vi "Send to Server.vi"() -> ()   [LabVIEW 2016]
uses:
  AE Data.ctl
  Array AE Data.ctl
  <vilib>/httpClient/POSTBuffer.vi
  <vilib>/Utility/error.llb/Error Cluster From Error Code.vi
  <vilib>/ErrorRing/Error Ring.xnode
  <vilib>/httpClient/LabVIEWHTTPClient.lvlib
panel:
  out "error out 2":errorcluster
  in  "Tab Control":enum32{"Update My Details", "Debug"}(tab)
  in  "STOP":bool
  in  "Update":bool
  in  "AE":T1
  out "error out":errorcluster
  out "Array of AEs":T2=[{"Name"="Peng", "Go?"=TRUE, "Which batch?"=enum."Anything"}, {"Name"="Xue Sheng", "Go?"=TRUE, "Which batch?"=enum."Anything"}, {"Name"="Denny", "Go?"=TRUE, "Which batch?"=enum."Anything"}, {"Name"="Wilbur", "Go?"=TRUE, "Which batch?"=enum."Anything"}, {"Name"="Hafiz", "Go?"=TRUE, "Which batch?"=enum."Anything"}, {"Name"="James", "Go?"=TRUE, "Which batch?"=enum."Anything"}, {"Name"="Sharath", "Go?"=TRUE, "Which batch?"=enum."Anything"}, {"Name"="Habib", "Go?"=TRUE, "Which batch?"=enum."Anything"}, {"Name"="Stephen", "Go?"=TRUE, "Which batch?"=enum."Anything"}]
  in  "Get List":bool
  in  "url":string="http://10.155.16.37:8002/AELunch/Send"
  out "body":string
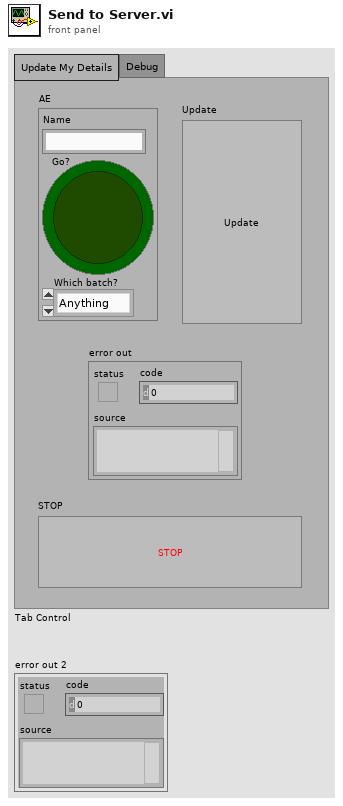
[diagram p1: front panel]
types:
  T1 = typedef "AE Data.ctl" = cluster{"Name":string, "Go?":bool, "Which batch?":enum16{"Anything", "First", "Second"}}
  T2 = typedef "Array AE Data.ctl" = T1[]
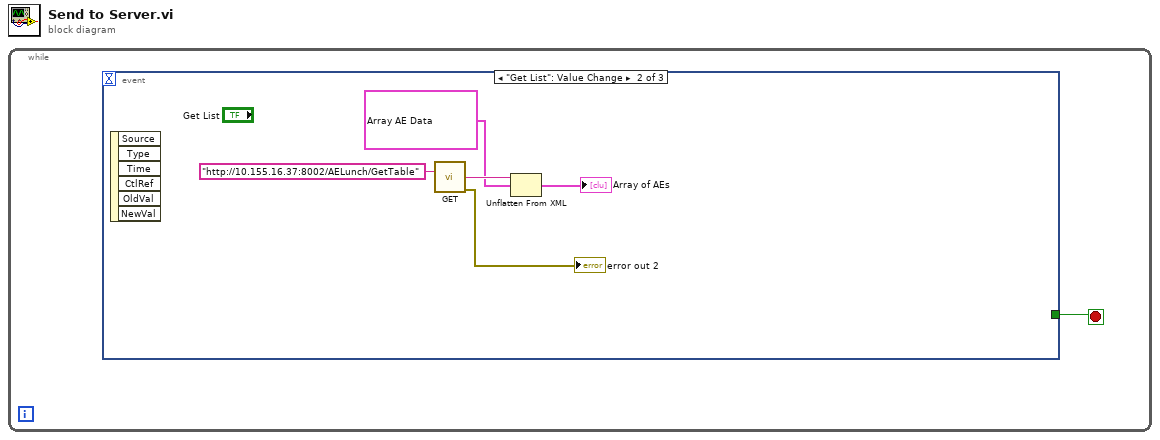
[diagram p0: block diagram]
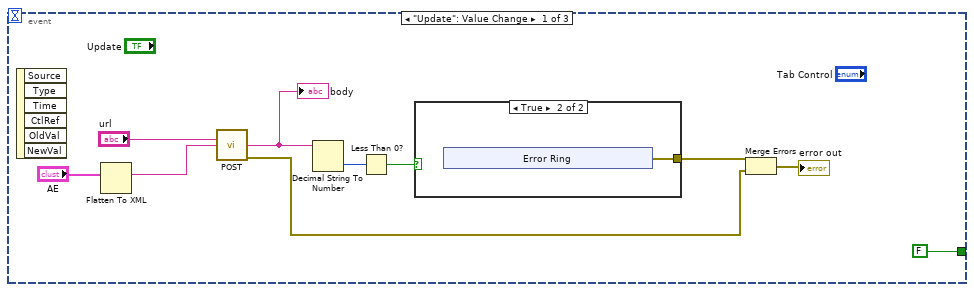
[diagram p2: hidden frame]
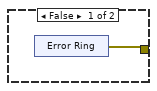
[diagram p3: hidden frame]
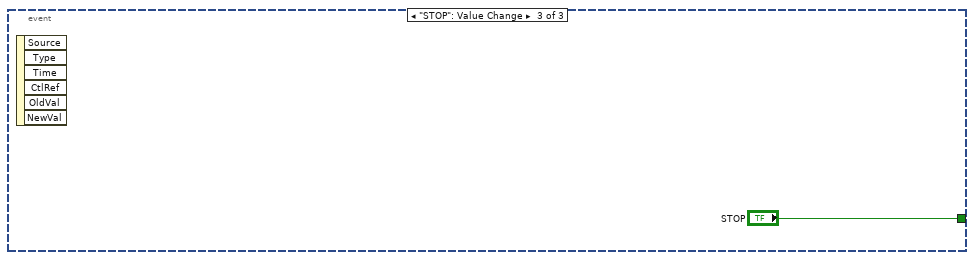
[diagram p4: hidden frame]
diagram:
  n1 = while {
    stop <- w1 stop-if-true
    n2 = event shown="[1] \"Get List\": Value Change" {
      selector: _ -> [_ _ _]
      dyn-events: _ -> [_ _ _]
      timeout: _ -> [_ _ _]
      tunnel: [FALSE _ "STOP"] -> w1
      event "Update": Value Change {
        n3 = event-data() -> ()  [unwired: 1 in, 6 out]
        n4 = Flatten To XML(anything="AE") -> (xml string=w9:string)
        n5 = call-poly <vilib>:"POST.vi"("url"="url", "buffer"=w9) -> ("body"=w8:string, "error out"=w4:errorcluster)  [unwired: 10 in, 2 out]
        "body" <- w8
        n6 = Decimal String To Number(string=w8) -> (number=w7:i32)  [unwired: 2 in, 1 out]
        n7 = Less Than 0?(x=w7) -> (x < 0?=w6:bool)
        n8 = case shown="True" w6 {
          tunnel: [w12 w14] -> w5
          frame False {
            n9 = xnode "Error Ring"() -> ("error out"=w12:errorcluster)
          }
          frame True {
            n10 = xnode "Error Ring"() -> ("error out"=w14:errorcluster)
          }
        }
        n11 = Merge Errors(w5, w4) -> (→"error out":errorcluster)
      }
      event "Get List": Value Change {
        n12 = event-data() -> ()  [unwired: 1 in, 6 out]
        n13 = call <vilib>:"GET.vi"("url"="http://10.155.16.37:8002/AELunch/GetTable") -> ("body"=w23:string, "error out"=→"error out 2":errorcluster)  [unwired: 11 in, 2 out]
        n14 = Unflatten From XML(xml string=w23, type=T2 [{"Name"="Peng", "Go?"=TRUE, "Which batch?"=enum."Anything"}, {"Name"="Xue Sheng", "Go?"=TRUE, "Which batch?"=enum."Anything"}, {"Name"="Denny", "Go?"=TRUE, "Which batch?"=enum."Anything"}, {"Name"="Wilbur", "Go?"=TRUE, "Which batch?"=enum."Anything"}, {"Name"="Hafiz", "Go?"=TRUE, "Which batch?"=enum."Anything"}, {"Name"="James", "Go?"=TRUE, "Which batch?"=enum."Anything"}, {"Name"="Sharath", "Go?"=TRUE, "Which batch?"=enum."Anything"}, {"Name"="Habib", "Go?"=TRUE, "Which batch?"=enum."Anything"}, {"Name"="Stephen", "Go?"=TRUE, "Which batch?"=enum."Anything"}] ("Array of AEs 2")) -> (value=→"Array of AEs":T2)  [unwired: 1 in, 1 out]
      }
      event "STOP": Value Change {
        n15 = event-data() -> ()  [unwired: 1 in, 6 out]
      }
    }
  }
